vi "SLM Initialize 640.vi"(4 "error in (no error)":errorcluster, 7 "VISA Resource Name":refnum<visa-resource-name>) -> (0 "error out":errorcluster, 1 "Dual":bool, 2 "Number of Pixels":u16, 3 "dup VISA resource name":refnum<visa-resource-name>)   [LabVIEW 2022 SP3]
panel:
  out "Serial Number":string
  out "Hardware Rev.":string
  out "Firmware Rev.":string
  out "QUERY":string
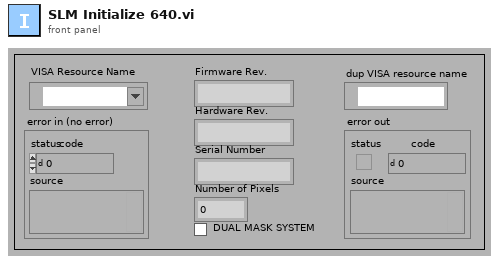
[diagram p1: front panel]
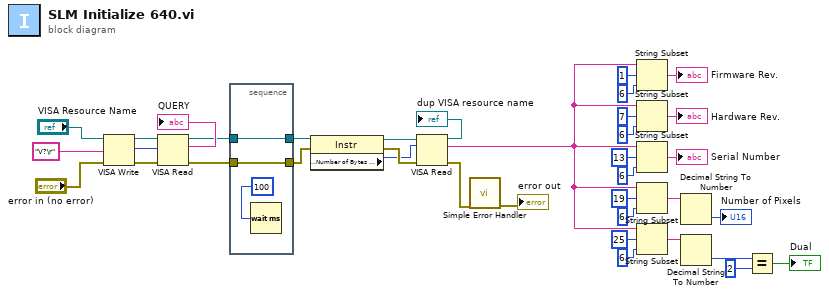
[diagram p0: block diagram]
diagram:
  n1 = VISA Write(VISA resource name="VISA Resource Name", write buffer="V?\r" ("write buffer (\"\")"), error in (no error)="error in (no error)") -> (VISA resource name out=w34:refnum<visa-resource-name>, return count=w35:u32, error out=w33:errorcluster)
  n2 = VISA Read(VISA resource name=w34, byte count=w35, error in (no error)=w33) -> (VISA resource name out=w4:refnum<visa-resource-name>, read buffer=→"QUERY":string, error out=w2:errorcluster)  [unwired: 1 out]
  n3 = stacked-sequence {
    tunnel: w4 -> [w39]
    tunnel: [w39] -> w3
    tunnel: w2 -> [w38]
    tunnel: [w38] -> w1
    frame #0 {
      n4 = Wait (ms)(milliseconds to wait=u32 100) -> ()  [unwired: 1 out]
    }
  }
  n5 = property class="Instr"(reference=w3, error in=w1) -> (reference out=w29:refnum<visa-resource-name>, error out=w28:errorcluster, "Serial Settings:Number of Bytes at Serial Port"=w27:u32)
  n6 = VISA Read(VISA resource name=w29, byte count=w27, error in (no error)=w28) -> (VISA resource name out=→"dup VISA resource name":refnum<visa-resource-name>, read buffer=w11:string, error out=w25:errorcluster)  [unwired: 1 out]
  n7 = call <vilib>:"Simple Error Handler.vi"("error in (no error)"=w25) -> ("error out"=→"error out":errorcluster)  [unwired: 4 in, 4 out]
  n8 = String Subset(string=w11, offset (0)=1, length (rest)=6 ("length (rest)")) -> (substring=→"Firmware Rev.":string)
  n9 = String Subset(string=w11, offset (0)=7, length (rest)=6 ("length (rest)")) -> (substring=→"Hardware Rev.":string)
  n10 = String Subset(string=w11, offset (0)=13, length (rest)=6 ("length (rest)")) -> (substring=→"Serial Number":string)
  n11 = String Subset(string=w11, offset (0)=19, length (rest)=6 ("length (rest)")) -> (substring=w10:string)
  n12 = String Subset(string=w11, offset (0)=25, length (rest)=6 ("length (rest)")) -> (substring=w9:string)
  n13 = Decimal String To Number(string=w10) -> (number=→"Number of Pixels":i32)  [unwired: 2 in, 1 out]
  n14 = Decimal String To Number(string=w9) -> (number=w7:i32)  [unwired: 2 in, 1 out]
  n15 = Equal?(x=w7, y=2) -> (x = y?=→"Dual":bool)
